vi "VA CoAP - Message - Option Insert - 23 Block2.vi"(0 "CoAP Message IN":string, 5 "Current Option Delta":u8, 7 "NUM (incremental block number within original data)":u8, 9 "M (more blocks flag)":u8(ring)=1 items=["No", "Yes"], 11 "SZX (block size)":u8(ring)=1 items=["16", "32", "64", "128", "256", "512", "1024"]) -> (4 "CoAP Message OUT":string, 6 "New Option Delta":u8)   [LabVIEW 2020]
panel:
  out "x .or. y?":bool[](array[boolean])
  out "Message Length":bool[](array[boolean])
  out "NUM":bool[](array[boolean])
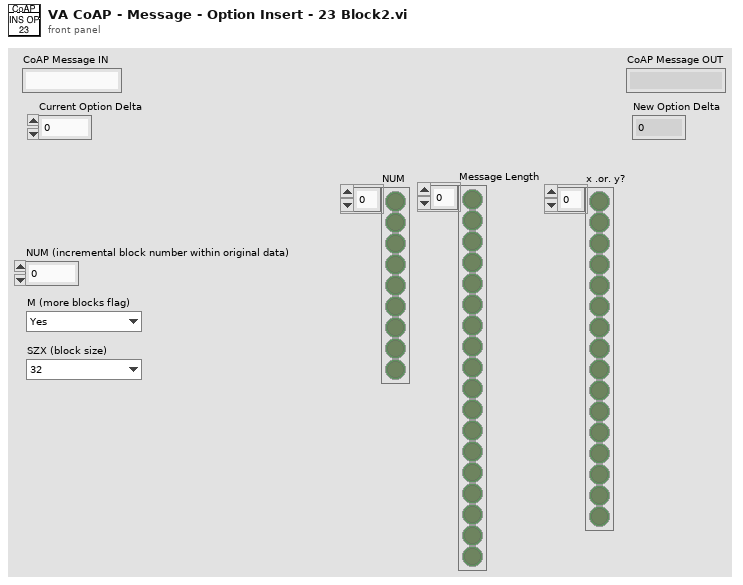
[diagram p1: front panel]
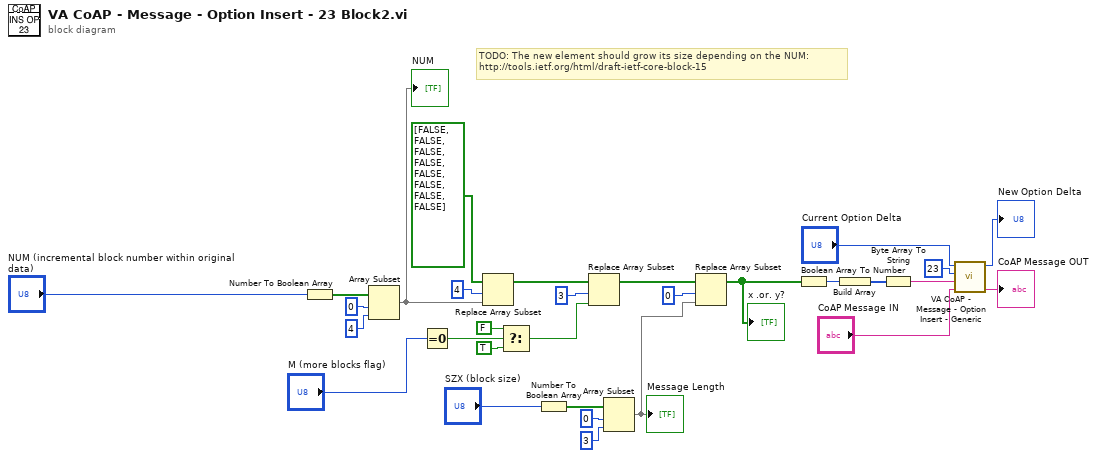
[diagram p0: block diagram]
diagram:
  # "TODO: The new element should grow its size depending on the NUM:\nhttp://tools.ietf.org/html/draft-ietf-core-block-15"
  n1 = Number To Boolean Array(number="NUM (incremental block number within original data)") -> (Boolean array=w16:bool[])
  n2 = Array Subset(array=w16, index=0, length=4) -> (w13:bool[])
  "NUM" <- w13
  n3 = Equal To 0?(x="M (more blocks flag)") -> (x = 0?=w8:bool)
  n4 = Replace Array Subset(array=bool[] [FALSE, FALSE, FALSE, FALSE, FALSE, FALSE, FALSE, FALSE], new element=w13, index=4) -> (w11:bool[])
  n5 = Select(t=FALSE, s=w8, f=TRUE) -> (s? t:f=w5:bool)
  n6 = Number To Boolean Array(number="SZX (block size)") -> (Boolean array=w24:bool[])
  n7 = Replace Array Subset(array=w11, new element=w5, index=3) -> (w10:bool[])
  n8 = Array Subset(array=w24, index=0, length=3) -> (w20:bool[])
  "Message Length" <- w20
  n9 = Replace Array Subset(array=w10, new element=w20, index=0) -> (w21:bool[])
  "x .or. y?" <- w21
  n10 = Boolean Array To Number(Boolean array=w21) -> (number=w25:u32)
  n11 = Build Array(w25) -> (w26:u32[])
  n12 = Byte Array To String(unsigned byte array=w26) -> (string=w3:string)
  n13 = call "VA CoAP - Message - Option Insert - Generic.vi"("CoAP Message IN"="CoAP Message IN", "New Message Element"=w3, "Current Delta on Evaluation"=u8 23 ("Current Option Delta"), "Current Option Delta in"="Current Option Delta") -> ("CoAP Message OUT"=→"CoAP Message OUT":string, "Current Option Delta out"=→"New Option Delta":u8)  [unwired: 6 in]
